vi "Read IO Task.vi"(8 "error in (no error)":errorcluster, 10 "Task Name":string, 11 "Gantry in":refnum<class "Gantry.lvclass">) -> (0 "error out":errorcluster, 2 "task/channels in":refnum<k21>, 3 "Gantry out":refnum<class "Gantry.lvclass">)   [LabVIEW 2017, in "Gantry.lvclass"]
uses:
  Gantry.lvclass
  Gantry.lvclass/Gantry.ctl
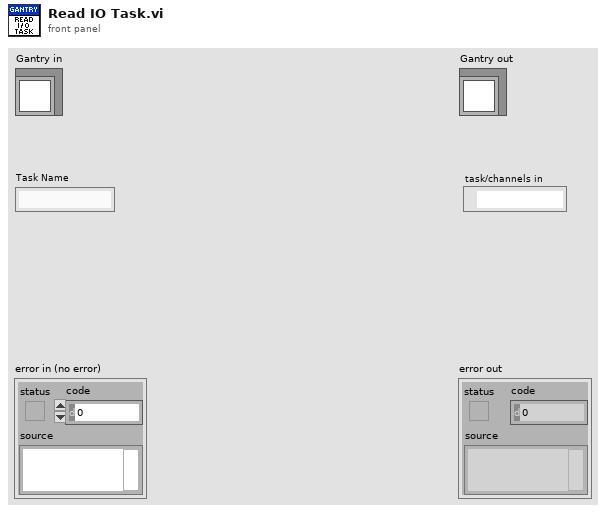
[diagram p1: front panel]
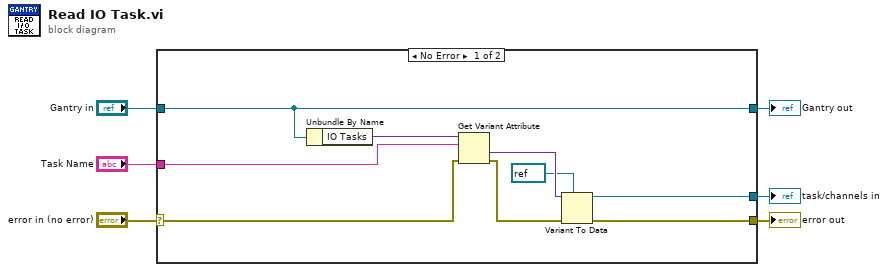
[diagram p0: block diagram]
diagram:
  n1 = case shown="No Error" "error in (no error)" {
    selector: "error in (no error)" -> [w12 w17]
    tunnel: [w9 w17] -> w5
    tunnel: [w15 w16] -> w3
    tunnel: "Gantry in" -> [w15 w16]
    tunnel: "Task Name" -> [w13 _]
    tunnel: [w7 _] -> w1
    frame No Error {
      n2 = Unbundle By Name(w15) -> ("IO Tasks"=w14:variant)
      n3 = Get Variant Attribute(Variant=w14, name=w13, error in=w12) -> (value=w11:variant, error out=w10:errorcluster)  [unwired: 1 in, 2 out]
      n4 = Variant To Data(error in=w10, type=refnum<k21> refnum ("task/channels in"), Variant=w11) -> (data=w7:refnum<k21>, error out=w9:errorcluster)
    }
    frame Error {
    }
  }
  "error out" <- w5
  "Gantry out" <- w3
  "task/channels in" <- w1
